vi "TCP schreiben.vi"(8 "error in":errorcluster caption="error out", 10 "String":string, 11 "connection ID":refnum<k5>) -> (0 "error out":errorcluster, 2 "Verknüpfter String":string, 3 "connection ID":refnum<k5>)   [LabVIEW 2020, in "AK-Schnittstelle.lvlib" / "AK TCP.lvlib"]
uses:
  AK TCP.lvlib
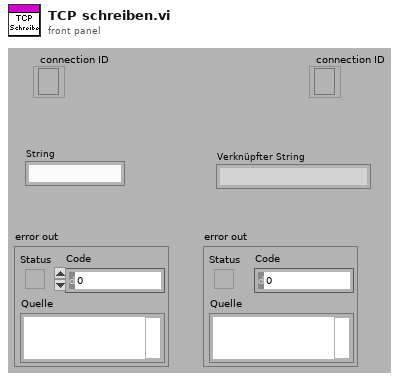
[diagram p1: front panel]
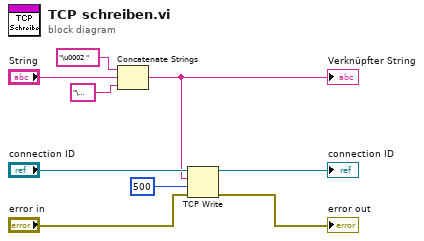
[diagram p0: block diagram]
diagram:
  n1 = Concatenate Strings("\u0002 " ("String"), "String", "\u0003" ("String")) -> (w1:string)
  "Verknüpfter String" <- w1
  n2 = TCP Write(connection ID="connection ID", data in=w1, error in (no error)="error in", 9:500 ("Timeout in ms (25000)")) -> (connection ID out=→"connection ID":refnum<k5>, error out=→"error out":errorcluster)  [unwired: 1 out]
